vi "Calcul Aire Spectre.vi"(8 "error in (no error)":errorcluster caption="entrée d'erreur (pas d'erreur)", 10 "Data Queue":T1, 11 "UI SA en entrée":refnum<class "UI SmarAct.lvclass">) -> (0 "error out":errorcluster caption="sortie d'erreur", 1 "Zoom Spectre":cluster{dbl[], dbl[]}, 2 "Spectre":T1, 3 "UI SA en sortie":refnum<class "UI SmarAct.lvclass">, 4 "PosX.Curs-1":dbl, 5 "PosX.Curs-0":dbl, 6 "Aire":dbl)   [LabVIEW 2024, in "UI SmarAct.lvclass"]
uses:
  UI SmarAct.lvclass
  UI SmarAct.lvclass/UI SmarAct.ctl
  <vilib>/Analysis/8numeric.llb/1D Numeric Integration.vi
  <vilib>/Analysis/NI_AALPro.lvlib
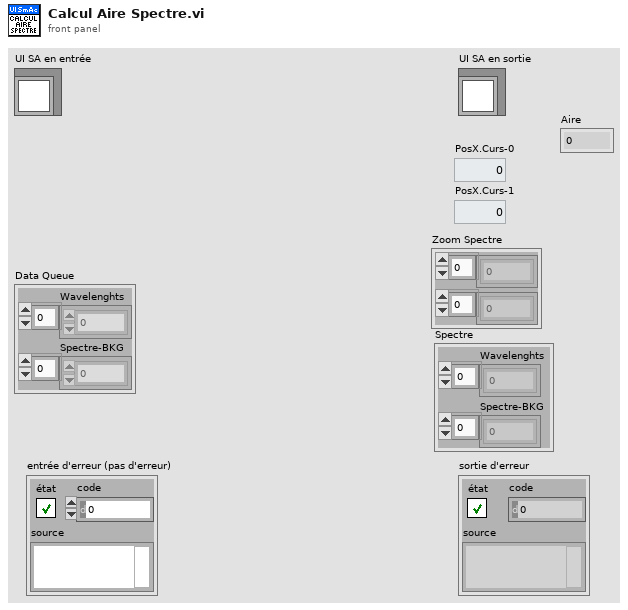
[diagram p1: front panel]
types:
  T1 = cluster{"Wavelenghts":dbl[], "Spectre-BKG":dbl[]}
  T2 = typedef "LVPointDoubleTypeDef.ctl" = cluster{"Cursor X":dbl, "Cursor Y":dbl}
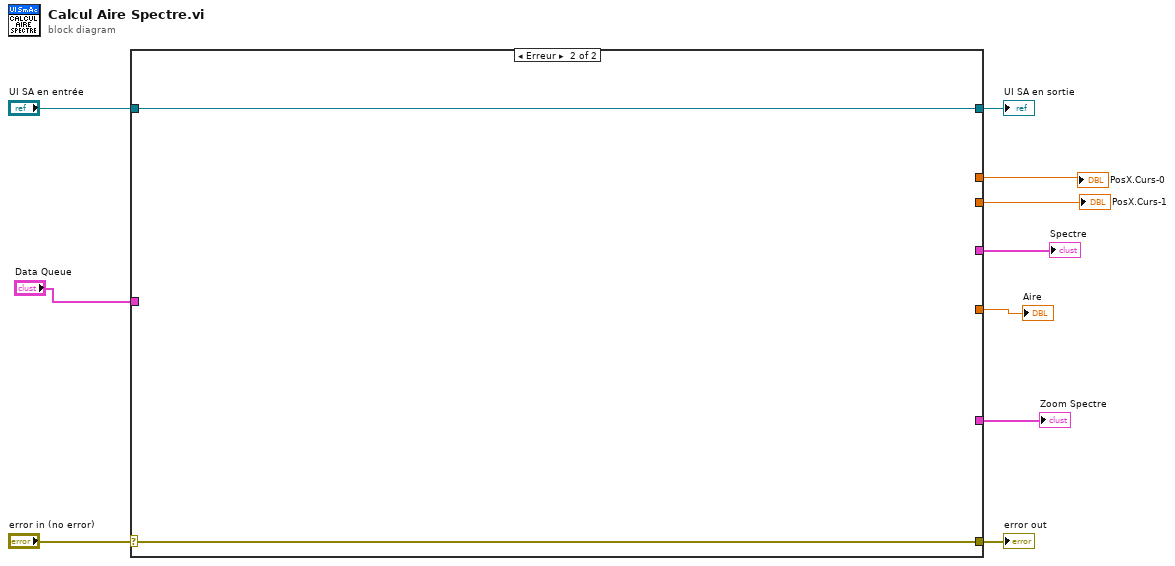
[diagram p0: block diagram]
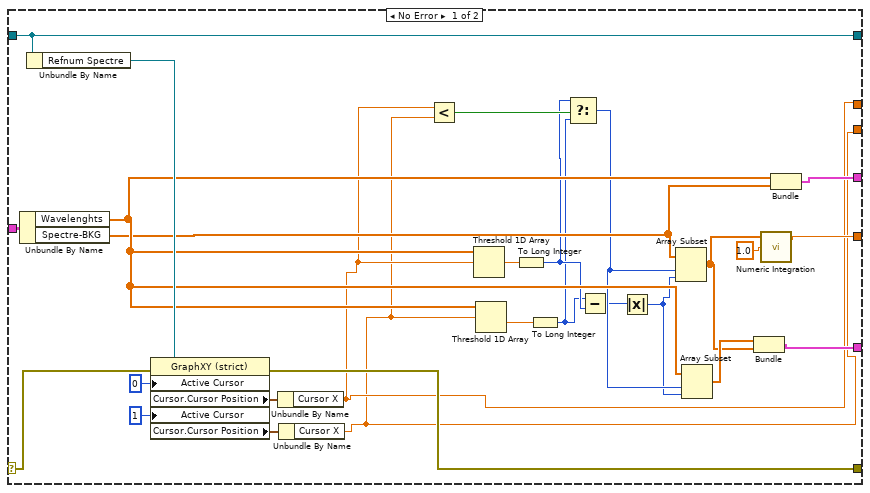
[diagram p2: hidden frame]
diagram:
  n1 = case shown="Erreur" "error in (no error)" {
    selector: "error in (no error)" -> [w27 w39]
    tunnel: [w26 w39] -> w9
    tunnel: [w33 w38] -> w7
    tunnel: "UI SA en entrée" -> [w33 w38]
    tunnel: [w14 _] -> w6
    tunnel: [w13 _] -> w5
    tunnel: [w24 _] -> w4
    tunnel: [w23 _] -> w3
    tunnel: "Data Queue" -> [w22 _]
    tunnel: [w19 _] -> w1
    frame No Error {
      n2 = Unbundle By Name(w22) -> ("Wavelenghts"=w21:dbl[], "Spectre-BKG"=w20:dbl[])
      n3 = Unbundle By Name(w33) -> ("Refnum Spectre"=w28:refnum<vi>)
      n4 = property class="GraphXY (strict)"(reference=w28, error in=w27, "Active Cursor"=u32 0 ("Curseur.Indice du curseur"), "Active Cursor"=u32 1 ("Curseur actif")) -> (error out=w26:errorcluster, "Cursor.Cursor Position"=w31:T2, "Cursor.Cursor Position"=w29:T2)  [unwired: 1 out]
      n5 = Unbundle By Name(w31) -> ("Cursor X"=w14:dbl)
      n6 = Unbundle By Name(w29) -> ("Cursor X"=w13:dbl)
      n7 = Less?(x=w14, y=w13) -> (x < y?=w18:bool)
      n8 = Threshold 1D Array(2:w14, 3:w21) -> (0:w35:dbl)  [unwired: 1 in]
      n9 = Threshold 1D Array(2:w13, 3:w21) -> (0:w34:dbl)  [unwired: 1 in]
      n10 = To Long Integer(number=w35) -> (32bit integer=w17:i32)
      n11 = To Long Integer(number=w34) -> (32bit integer=w15:i32)
      n12 = Select(t=w17, s=w18, f=w15) -> (s? t:f=w16:i32)
      n13 = Subtract(x=w15, y=w17) -> (x-y=w12:i32)
      n14 = Absolute Value(x=w12) -> (abs(x)=w11:i32)
      n15 = Array Subset(array=w20, index=w16, length=w11) -> (w25:dbl[])
      n16 = Array Subset(array=w21, index=w16, length=w11) -> (w37:dbl[])
      n17 = Bundle(w37, w25) -> (w23:cluster{dbl[], dbl[]})  [unwired: 1 in]
      n18 = call-poly <vilib>:"Numeric Integration.vi"("dt"=1.0, "Input Array"=w25) -> ("result"=w24:dbl)  [unwired: 1 in, 1 out]
      n19 = Bundle("Wavelenghts"=w21, "Spectre-BKG"=w20) -> (w19:T1)  [unwired: 1 in]
    }
    frame Error {
    }
  }
  "error out" <- w9
  "UI SA en sortie" <- w7
  "PosX.Curs-0" <- w6
  "PosX.Curs-1" <- w5
  "Aire" <- w4
  "Zoom Spectre" <- w3
  "Spectre" <- w1
